vi "SubVI_HP4263A_10kHz.vi"(4 "error in (no error)":errorcluster, 5 "averaging count (1)":i16=1 min=1 max=256 step=1, 6 "function (Z - Angle:0)":u16(ring) items=["Z - Angle", "R - X", "Y - Angle", "G - B", "CP - D", "CP - Q", "CP - G", "CS - D", "CS - Q", "CS - RS", "LP - D", "LP - Q", "LP - G", "LS - D", "LS - Q", "LS - RS", "LS - DCR (option 001 only)", "LP - DCR (option 001 only)", "L2 - N (option 001 only)", "L2 - M (option 001 only)", "L2 - R2 (option 001 only)"], 7 "VISA resource name":refnum<visa-resource-name>) -> (0 "error out":errorcluster, 1 "secondary reading":dbl format="%.5e", 2 "primary reading":dbl format="%.5e", 3 "status":u16)   [LabVIEW 2010]
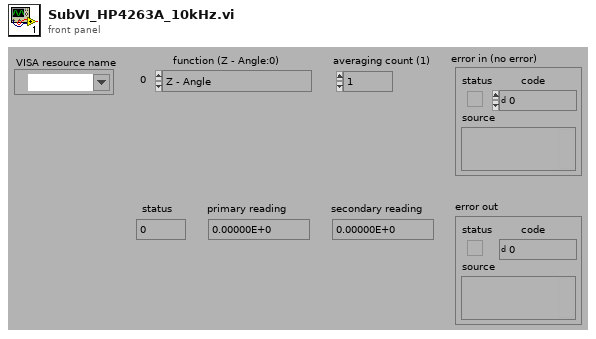
[diagram p1: front panel]
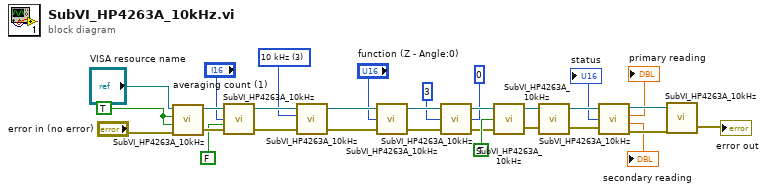
[diagram p0: block diagram]
diagram:
  w26 = u16 3 items=["100 Hz", "120 Hz", "1 kHz", "10 kHz", "20 kHz (option 002 ONLY)", "100 kHz"] ("frequency (100 Hz:0)")
  w21 = TRUE
  n1 = call "SubVI_HP4263A_10kHz.vi"("error in (no error)"="error in (no error)", "reset"=w21, "ID query"=w21, "VISA resource name"="VISA resource name") -> ("error out"=w19:errorcluster, "VISA session"=w18:refnum<visa-resource-name>)
  n2 = call "SubVI_HP4263A_10kHz.vi"("state (on:T)"=FALSE, "error in (no error)"=w19, "count (1)"="averaging count (1)", "VISA session"=w18) -> ("error out"=w29:errorcluster, "dup VISA session"=w27:refnum<visa-resource-name>)
  n3 = call "SubVI_HP4263A_10kHz.vi"("error in (no error)"=w29, "frequency (100 Hz:0)"=w26, "VISA session"=w27) -> ("error out"=w30:errorcluster, "dup VISA session"=w28:refnum<visa-resource-name>)  [unwired: 2 in]
  n4 = call "SubVI_HP4263A_10kHz.vi"("error in (no error)"=w30, "function (Z - Angle:0)"="function (Z - Angle:0)", "VISA session"=w28) -> ("error out"=w7:errorcluster, "dup VISA session"=w6:refnum<visa-resource-name>)  [unwired: 1 in]
  n5 = call "SubVI_HP4263A_10kHz.vi"("trigger delay (sec)"=0, "error in (no error)"=w7, "trigger source (int:0)"=3, "VISA session"=w6) -> ("error out"=w11:errorcluster, "dup VISA session"=w12:refnum<visa-resource-name>)
  n6 = call "SubVI_HP4263A_10kHz.vi"("error in (no error)"=w11, "initiate mode (cont:T)"=TRUE, "VISA session"=w12) -> ("error out"=w14:errorcluster, "dup VISA session"=w13:refnum<visa-resource-name>)  [unwired: 1 in]
  n7 = call "SubVI_HP4263A_10kHz.vi"("error in (no error)"=w14, "VISA session"=w13) -> ("error out"=w9:errorcluster, "dup VISA session"=w10:refnum<visa-resource-name>)
  n8 = call "SubVI_HP4263A_10kHz.vi"("VISA session"=w10, "error in (no error)"=w9) -> ("status"=→"status":u16, "dup VISA session"=w22:refnum<visa-resource-name>, "primary reading"=→"primary reading":dbl, "secondary reading"=→"secondary reading":dbl, "error out"=w23:errorcluster)  [unwired: 2 out]
  n9 = call "SubVI_HP4263A_10kHz.vi"("error in (no error)"=w23, "dup VISA session"=w22) -> ("error out"=→"error out":errorcluster)  [unwired: 1 in]
